vi "Set Status.vi"(8 "error in (no error)":errorcluster, 10 "Status":bool, 11 "FlipMir in":refnum<class "FlipMir.lvclass">) -> (0 "error out":errorcluster, 3 "FlipMir out":refnum<class "FlipMir.lvclass">)   [LabVIEW 2016, in "FlipMir.lvclass"]
uses:
  FlipMir.lvclass
  FlipMir.lvclass/FlipMir.ctl
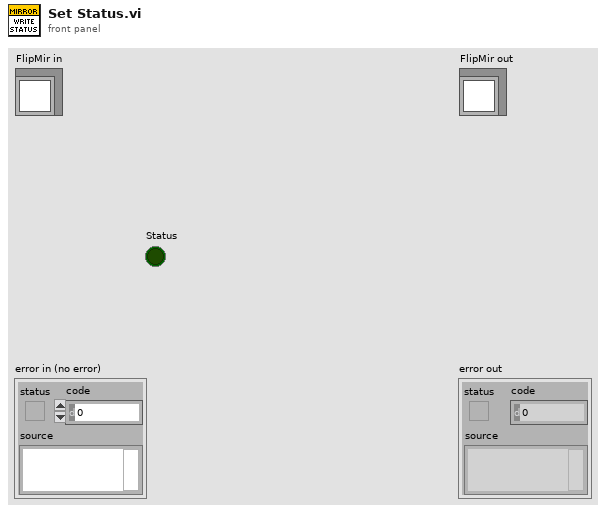
[diagram p1: front panel]
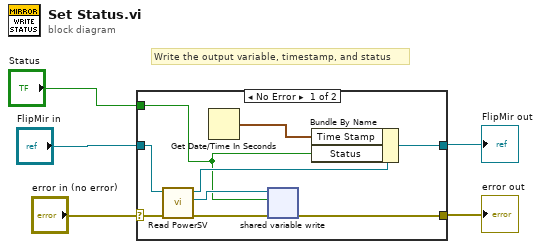
[diagram p0: block diagram]
diagram:
  # "Write the output variable, timestamp, and status"
  n1 = case shown="No Error" "error in (no error)" {
    selector: "error in (no error)" -> [w6 w16]
    tunnel: [w7 w16] -> w4
    tunnel: [w9 w15] -> w2
    tunnel: "FlipMir in" -> [w14 w15]
    tunnel: "Status" -> [w8 _]
    frame No Error {
      n2 = call-dynamic "Read PowerSV.vi"("error in (no error)"=w6, "FlipMir in"=w14) -> ("error out"=w10:errorcluster, "PowerSV"=w11:refnum<k21>, "FlipMir out"=w12:refnum<class "FlipMir.lvclass">)  [unwired: 7 in]
      n3 = Get Date/Time In Seconds() -> (seconds since 1Jan1904=w13:timestamp)
      n4 = shared-variable-write(w11, w10, w8) -> (w7:errorcluster)  [unwired: 1 out]
      n5 = Bundle By Name(cluster=w12, "Time Stamp"=w13, "Status"=w8) -> (w9:refnum<class "FlipMir.lvclass">)
    }
    frame Error {
    }
  }
  "error out" <- w4
  "FlipMir out" <- w2
